vi "Orca Flash Capture Scan Counter Cycles Steps.vi"(8 "Cycles Steps Tracker":T1) -> (0 "Cycles Steps Tracker Out":T1, 2 "Change Cycle?":bool, 3 "Done?":bool)   [LabVIEW 2020]
uses:
  Orca Flash Capture Manager Controls/Orca Flash Capture Cycle Step Count.ctl
  Orca Flash Capture Manager Controls/Orca Flash Switch Cycles Steps.ctl
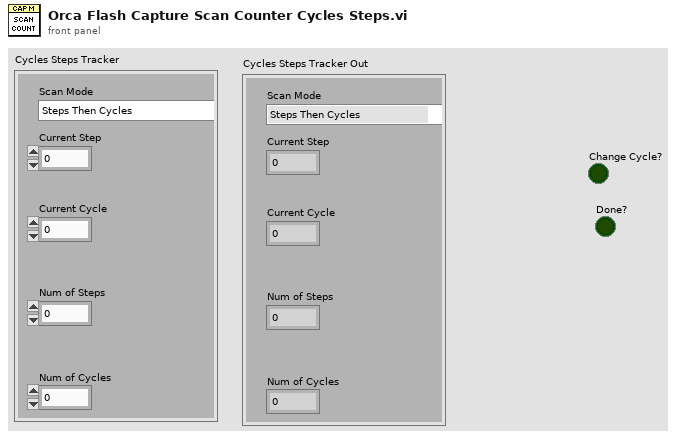
[diagram p1: front panel]
types:
  T1 = typedef "Orca Flash Capture Cycle Step Count.ctl" = cluster{"Scan Mode":T2, "Current Step":u16, "Current Cycle":u16, "Num of Steps":u16, "Num of Cycles":u16}
  T2 = typedef "Orca Flash Switch Cycles Steps.ctl" = enum16{"Steps Then Cycles", "Cycles Then Steps"}
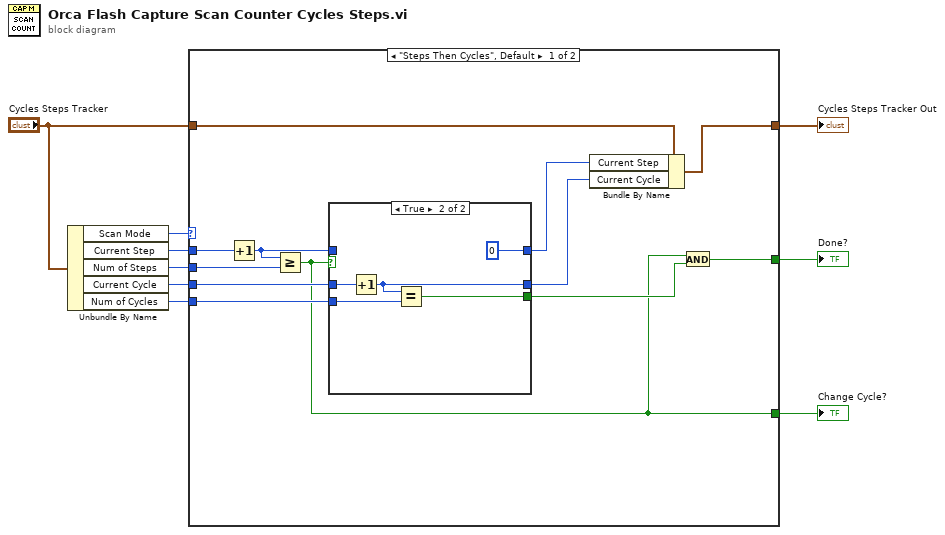
[diagram p0: block diagram]
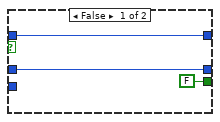
[diagram p2: hidden frame]
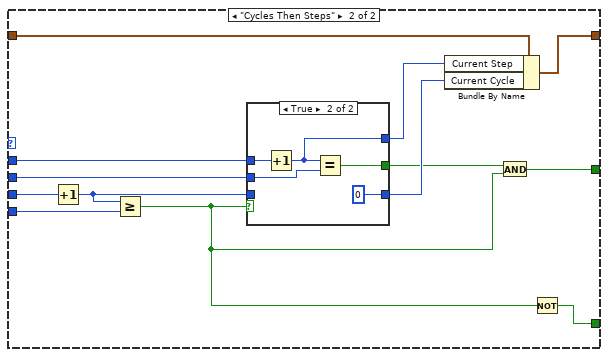
[diagram p3: hidden frame]
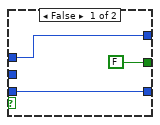
[diagram p4: hidden frame]
diagram:
  n1 = Unbundle By Name("Cycles Steps Tracker") -> ("Scan Mode"=w9:T2, "Current Step"=w7:u16, "Num of Steps"=w6:u16, "Current Cycle"=w5:u16, "Num of Cycles"=w4:u16)
  n2 = case shown="\"Steps Then Cycles\", Default" w9 {
    tunnel: "Cycles Steps Tracker" -> [w19 w40]
    tunnel: w7 -> [w21 w42]
    tunnel: w6 -> [w20 w36]
    tunnel: w5 -> [w17 w35]
    tunnel: w4 -> [w16 w41]
    tunnel: [w13 w32] -> w2
    tunnel: [w10 w30] -> w3
    tunnel: [w18 w37] -> w1
    frame "Steps Then Cycles", Default {
      n3 = Increment(x=w21) -> (x+1=w15:u16)
      n4 = Greater Or Equal?(x=w15, y=w20) -> (x >= y?=w10:bool)
      n5 = case shown="True" w10 {
        tunnel: w17 -> [w22 w29]
        tunnel: w16 -> [_ w28]
        tunnel: w15 -> [w24 _]
        tunnel: [w24 u16 0] -> w14
        tunnel: [FALSE w26] -> w12
        tunnel: [w22 w25] -> w11
        frame False {
        }
        frame True {
          n6 = Increment(x=w29) -> (x+1=w25:u16)
          n7 = Equal?(x=w25, y=w28) -> (x = y?=w26:bool)
        }
      }
      n8 = Bundle By Name(cluster=w19, "Current Step"=w14, "Current Cycle"=w11) -> (w18:T1)
      n9 = And(x=w10, y=w12) -> (x .and. y?=w13:bool)
    }
    frame "Cycles Then Steps" {
      n10 = Increment(x=w35) -> (x+1=w34:u16)
      n11 = Greater Or Equal?(x=w34, y=w41) -> (x >= y?=w31:bool)
      n12 = case shown="True" w31 {
        tunnel: w42 -> [w43 w50]
        tunnel: w36 -> [_ w46]
        tunnel: [FALSE w49] -> w33
        tunnel: w34 -> [w44 _]
        tunnel: [w44 u16 0] -> w38
        tunnel: [w43 w47] -> w39
        frame False {
        }
        frame True {
          n13 = Increment(x=w50) -> (x+1=w47:u16)
          n14 = Equal?(x=w47, y=w46) -> (x = y?=w49:bool)
        }
      }
      n15 = Bundle By Name(cluster=w40, "Current Step"=w39, "Current Cycle"=w38) -> (w37:T1)
      n16 = And(x=w33, y=w31) -> (x .and. y?=w32:bool)
      n17 = Not(x=w31) -> (.not. x?=w30:bool)
    }
  }
  "Change Cycle?" <- w3
  "Done?" <- w2
  "Cycles Steps Tracker Out" <- w1
